vi "StageTest3.vi"() -> ()   [LabVIEW 2020]
uses:
  StageOptions.ctl
  SettingCtrlOptions.ctl
  PosCtrlOptions.ctl
  libximc.lvlib
  <instrlib>/_niInstr/Basic Elements/v1/FPGA/niInstr Basic Elements v1 FPGA.lvlib
panel:
  out "Y Maximum":dbl
  out "X Max Stage":dbl=220.0 format="%#_13g"
  in  "Move Step":dbl=1.0
  in  "Start Stage":bool
  in  "Speed Control (mm/s)":sgl(slide)=1.0 min=0.1 scale=0.1..5.0
  out "Y Step Size":sgl format="%#.2g"
  out "X Step Size":sgl format="%#.2g"
  in  "Scan Mode":enum16{"Raster", "Serpentine"}(ring)
  out "Controller Open?":bool
  in  "Y Position Abs":dbl caption="Y Position"
  in  "X Position Abs":dbl caption="X Position"
  in  "Move to Start":bool
  out "Move Step halved":dbl=1.0
  in  "Stop Stage":bool
  in  "Outline":bool
  in  "Stop Motion":bool
  in  "Right":bool
  in  "Left":bool
  in  "Down":bool
  in  "Up":bool
  in  "AbsMove":bool
  out "Moving?":bool
  in  "Zero":bool
  out "Y Position":dbl format="%#.3g"
  out "X Position":dbl format="%#.3g"
  out "Stage Position":cluster{sgl[], sgl[]}(graph) caption="XY Graph - Dark"
  in  "X Start":sgl
  in  "X End":sgl=10.0
  in  "Y Start":sgl
  in  "Y End":sgl=8.0
  in  "Y Step Size":sgl=0.5
  in  "X Step Size":sgl=0.5
  out "Line Count":i32=6
  out "Pixel Count":i32=6
  in  "Close Stage":bool
  in  "Machine Mode":T1(ring)=enum."Normal"
  out "Peripheral Coordis":sgl[][](array[numeric])=[[0.0, 0.0], [1.8, 0.0], [3.6, 0.0], [5.3999996, 0.0], [7.2, 0.0], [9.0, 0.0], [9.0, 2.0], [7.2, 2.0], [5.3999996, 2.0], [3.6, 2.0], [1.8, 2.0], [0.0, 2.0], [0.0, 4.0], [1.8, 4.0], [3.6, 4.0], [5.3999996, 4.0], [7.2, 4.0], [9.0, 4.0], [9.0, 6.0], [7.2, 6.0], [5.3999996, 6.0], [3.6, 6.0], [1.8, 6.0], [0.0, 6.0], [0.0, 8.0], [1.8, 8.0], [3.6, 8.0], [5.3999996, 8.0], [7.2, 8.0], [9.0, 8.0], [9.0, 10.0], [7.2, 10.0], [5.3999996, 10.0], [3.6, 10.0], [1.8, 10.0], [0.0, 10.0]]
  in  "Next Coordinate Index":i32
  out "Step Sizes":sgl[](array[numeric])
  out "Coordinate Array":sgl[][](array[numeric])
  out "IDs":i32[](array[numeric])
  out "Calibration":cluster{dbl, "MicrostepMode":u32}[](array[cluster])
  in  "EdgePt/nPixelMap":bool=TRUE
  in  "Correction Table Path (Hidden)":path
  out "Serial nos":u32[](array[numeric])
  out "Stage Status":T2
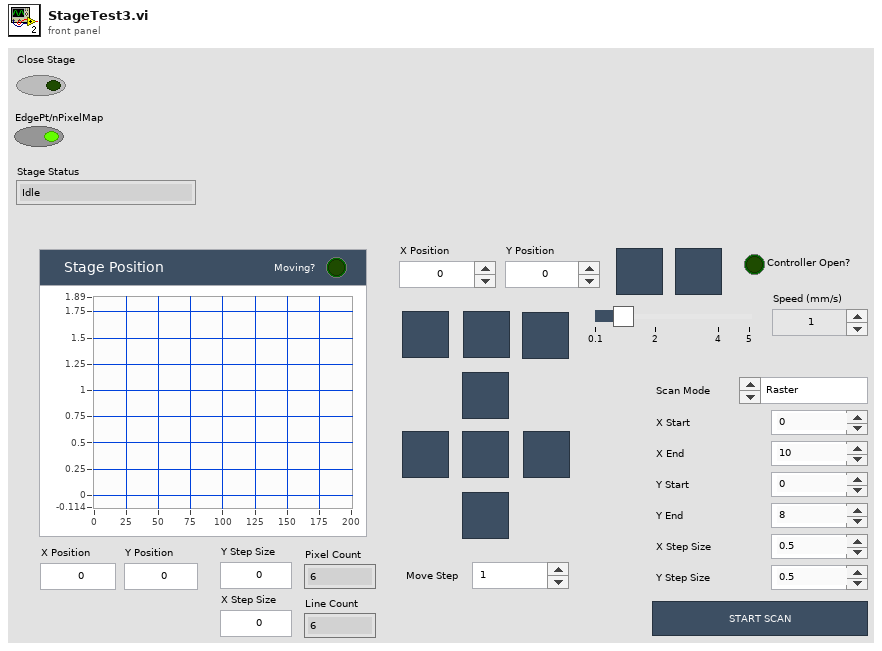
[diagram p1: front panel]
types:
  T1 = enum16{"Scanning Mode", "Perimeter Mode", "Normal"}
  T2 = typedef "StageOptions.ctl" = enum16{"Idle", "Init", "Set Speed", "GenerateMotionPoints", "Scan_Start", "Scan_MoveNext", "Scan_SyncSet", "Scan_Get Pos", "Scan_Complete", "Cmd_MoveAbs", "Cmd_CloseControllers", "Cmd_MoveUp", "Cmd_MoveDown", "Cmd_MoveLeft", "Cmd_MoveRight", "Cmd_MoveStart", "Cmd_MoveZero", "Cmd_GetPos", "Cmd_Stop", "Sync_On", "Sync_Off", "Stop Motion", "CloseApplication"}
  T3 = typedef "SettingCtrlOptions.ctl" = enum16{"Set X", "Set Y", "Set X and Y", "Get Settings", "None"}
  T4 = typedef "PosCtrlOptions.ctl" = enum16{"Move X", "Move Y", "Both X and Y", "Read Pos", "None"}
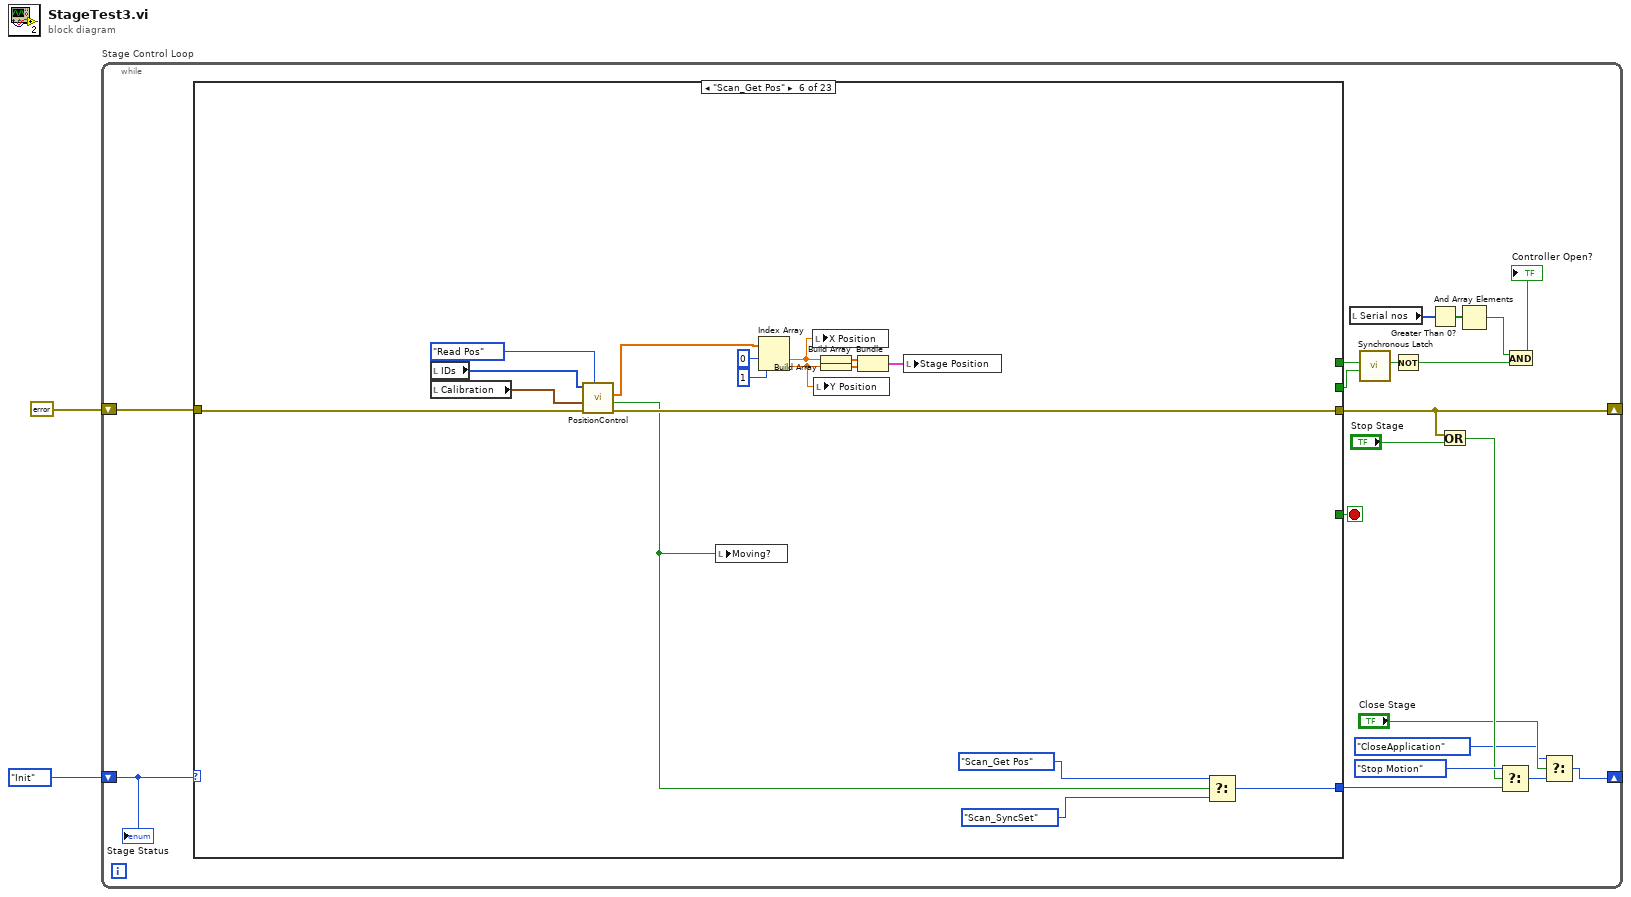
[diagram p0: block diagram]
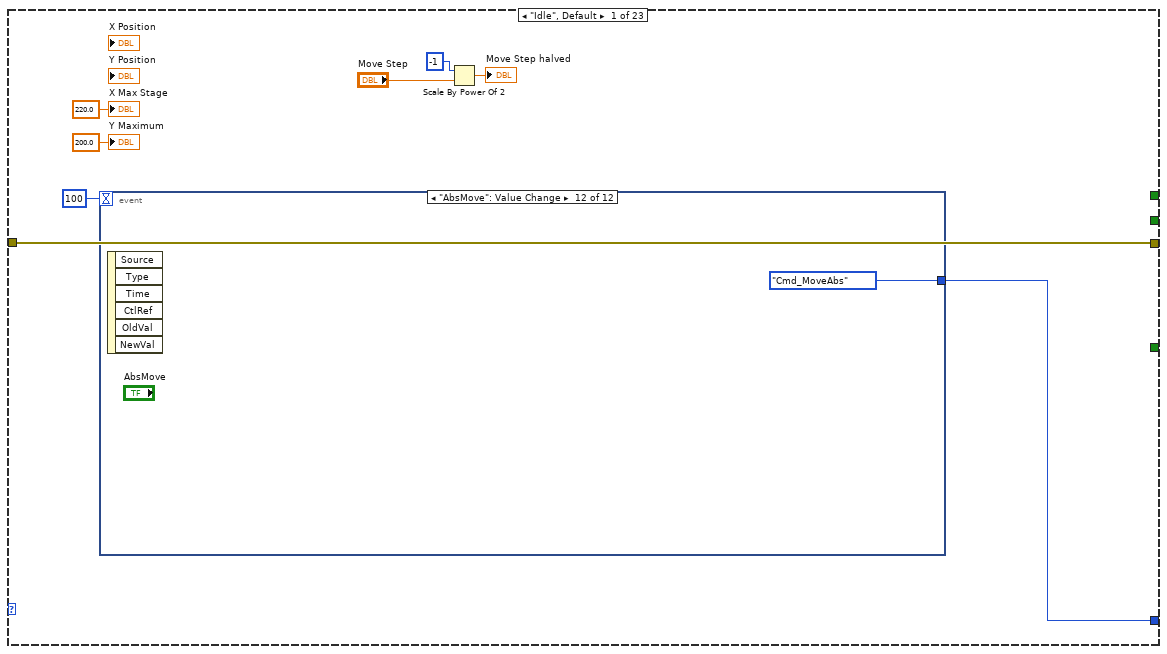
[diagram p2: hidden frame]
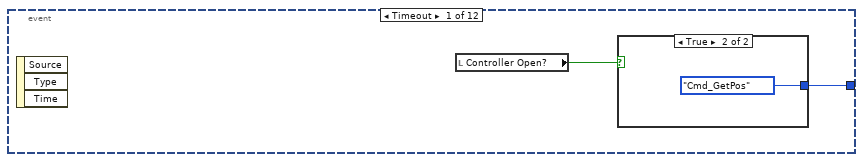
[diagram p3: hidden frame]
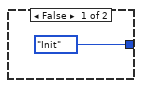
[diagram p4: hidden frame]
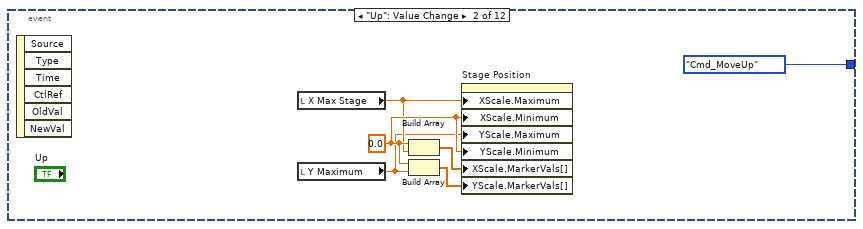
[diagram p5: hidden frame]
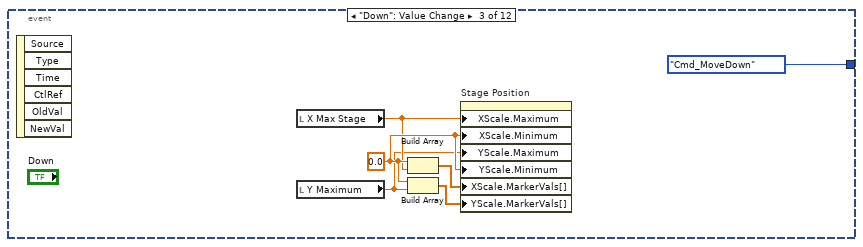
[diagram p6: hidden frame]
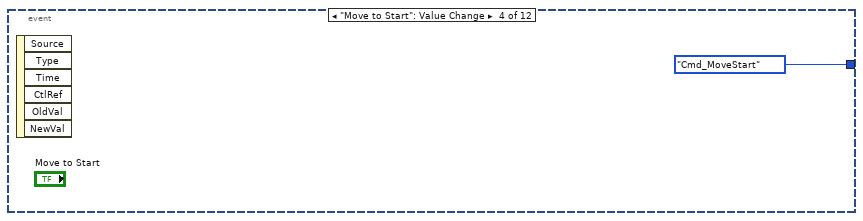
[diagram p7: hidden frame]
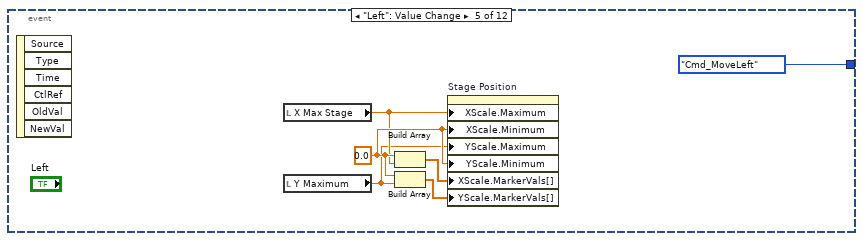
[diagram p8: hidden frame]
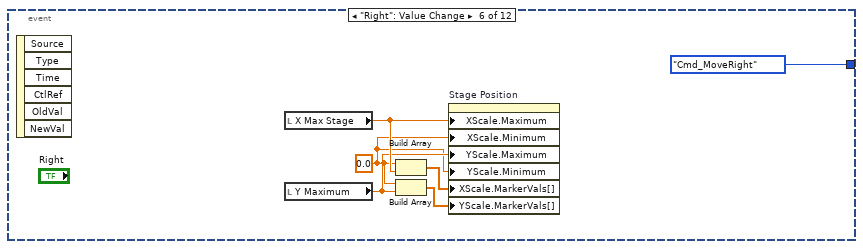
[diagram p9: hidden frame]
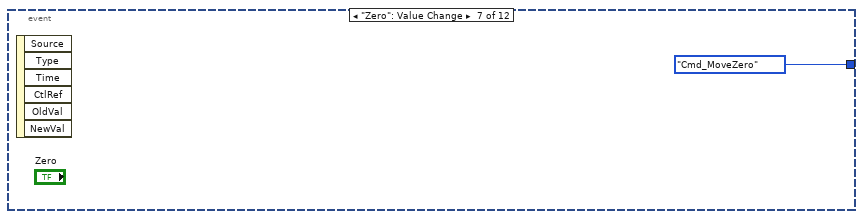
[diagram p10: hidden frame]
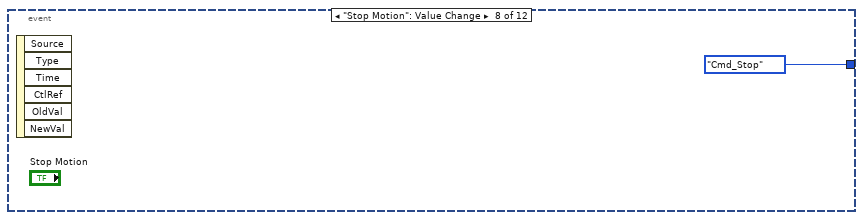
[diagram p11: hidden frame]
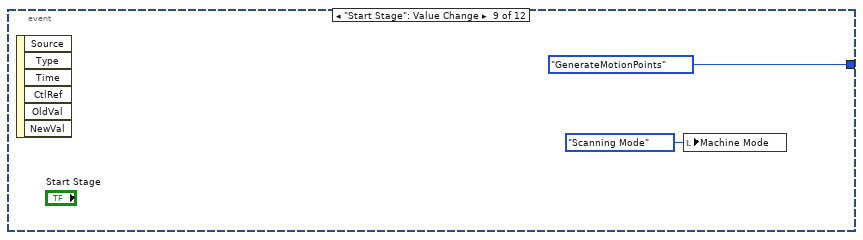
[diagram p12: hidden frame]
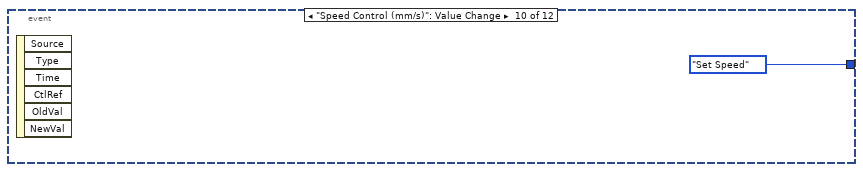
[diagram p13: hidden frame]
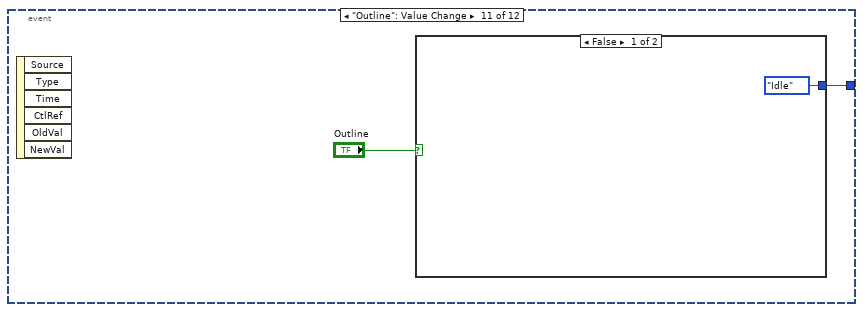
[diagram p14: hidden frame]
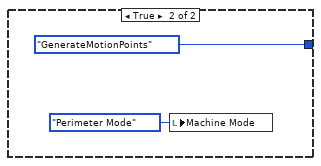
[diagram p15: hidden frame]
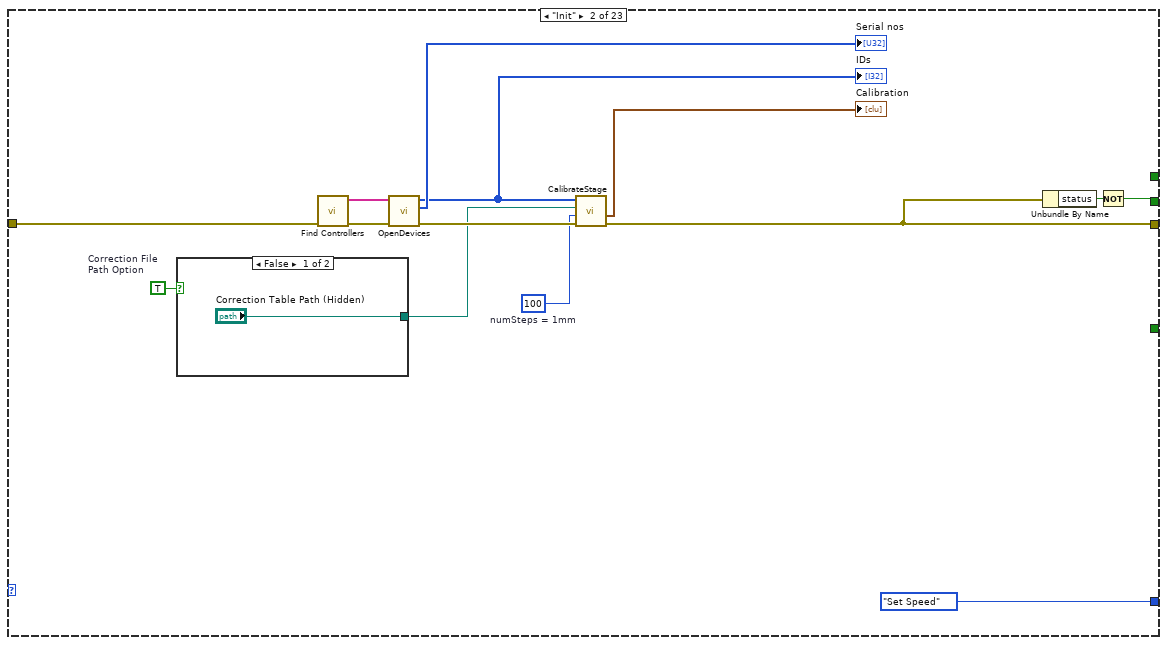
[diagram p16: hidden frame]
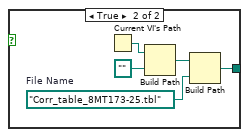
[diagram p17: hidden frame]
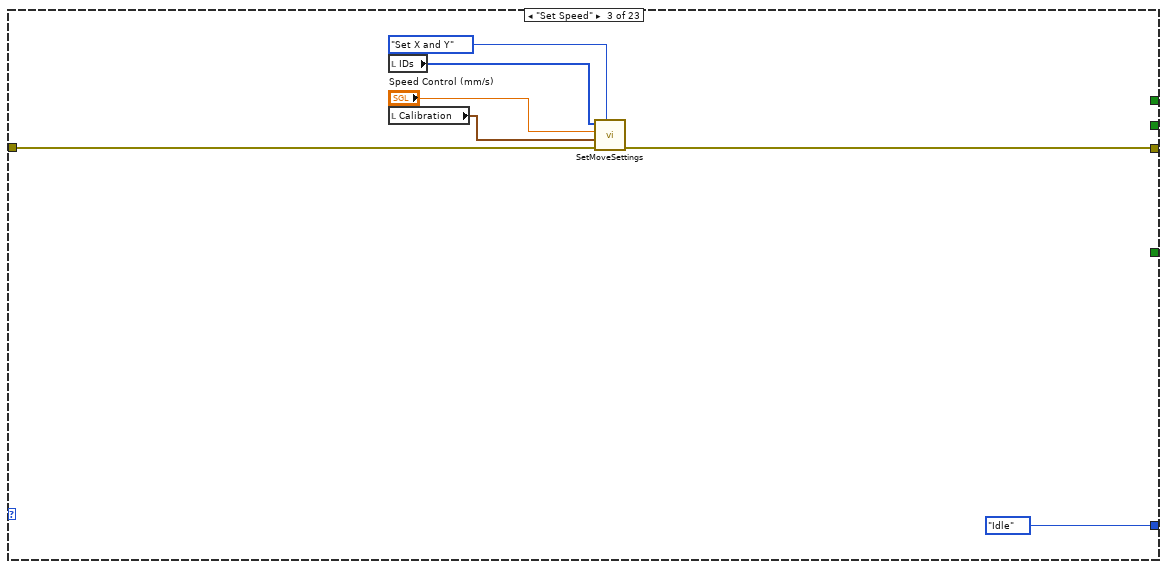
[diagram p18: hidden frame]
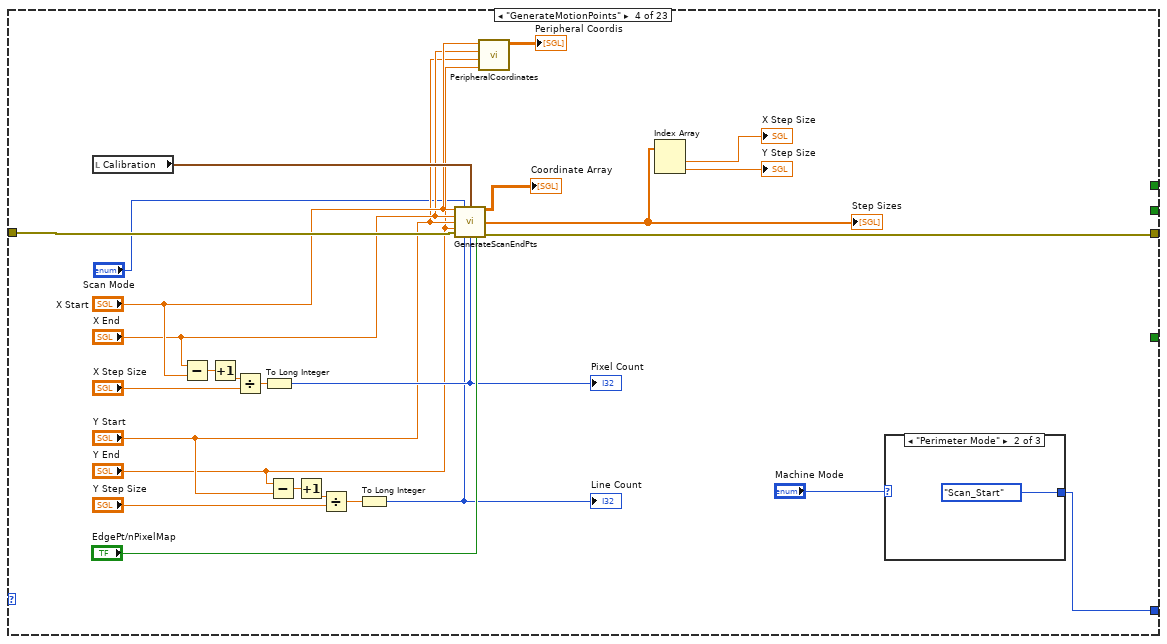
[diagram p19: hidden frame]
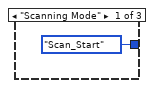
[diagram p20: hidden frame]
diagram:
  n1 = while "Stage Control Loop" {
    shift-right: [w11] -> _
    shift-left: StageOptions."Init" -> [w22]
    shift-right: [w19] -> _
    shift-left: errorcluster {"status"=FALSE, "code"=0, "source"=""} ("error out") -> [w20]
    stop <- w12 stop-if-true
    n2 = case shown="\"Scan_Get Pos\"" w22 {
      tunnel: [w30 w71 w94 w123 w137 w169 w183 w196 w237 w246 w255 w262 w273 w283 w293 w302 w310 w325 w331 w342 w351 w358 w368] -> w19
      tunnel: w20 -> [w30 w78 w95 w122 w143 w170 w184 w197 w238 w247 w256 w261 w274 w284 w294 w303 w311 w326 w330 w343 w352 w357 w367]
      tunnel: [w29 StageOptions."Set Speed" StageOptions."Idle" w103 StageOptions."Scan_Get Pos" w158 StageOptions."Scan_MoveNext" w193 StageOptions."Idle" StageOptions."Idle" StageOptions."Idle" StageOptions."Idle" StageOptions."Idle" StageOptions."Idle" StageOptions."Idle" StageOptions."Idle" StageOptions."Idle" StageOptions."Idle" StageOptions."Idle" StageOptions."Idle" StageOptions."Idle" StageOptions."Idle" StageOptions."Idle"] -> w17
      tunnel: [_ _ _ _ _ _ _ _ _ _ _ _ _ _ _ _ _ _ _ _ _ w354 w363] -> w15
      tunnel: [_ w72 _ _ _ _ _ _ _ _ _ _ _ _ _ _ _ _ _ _ _ _ _] -> w13
      tunnel: [_ _ _ _ _ _ _ _ _ _ _ _ _ _ _ _ _ _ _ _ _ _ w363] -> w12
      frame "Idle", Default {
        n3 = event shown="[11] \"AbsMove\": Value Change" {
          selector: _ -> [_ _ _ _ _ _ _ _ _ _ _ _]
          dyn-events: _ -> [_ _ _ _ _ _ _ _ _ _ _ _]
          timeout: 100 -> [_ _ _ _ _ _ _ _ _ _ _ _]
          tunnel: [w31 StageOptions."Cmd_MoveUp" StageOptions."Cmd_MoveDown" StageOptions."Cmd_MoveStart" StageOptions."Cmd_MoveLeft" StageOptions."Cmd_MoveRight" StageOptions."Cmd_MoveZero" StageOptions."Cmd_Stop" StageOptions."GenerateMotionPoints" StageOptions."Set Speed" w66 StageOptions."Cmd_MoveAbs"] -> w29
          event Timeout {
            n4 = event-data() -> ()  [unwired: 1 in, 3 out]
            n5 = local read "Controller Open?"() -> (w32:bool)
            n6 = case shown="True" w32 {
              tunnel: [StageOptions."Init" StageOptions."Cmd_GetPos"] -> w31
              frame False {
              }
              frame True {
              }
            }
          }
          event "Up": Value Change {
            w37 = 0.0 ("X Scale.Range:Minimum")
            n7 = event-data() -> ()  [unwired: 1 in, 6 out]
            n8 = local read "X Max Stage"() -> (w36:dbl)
            n9 = local read "Y Maximum"() -> (w35:dbl)
            n10 = Build Array(w37, w36) -> (w39:dbl[])
            n11 = Build Array(w37, w35) -> (w38:dbl[])
            n12 = property on="Stage Position" class="XYGraph (strict)"("XScale.Maximum"=w36, "XScale.Minimum"=w37, "YScale.Maximum"=w35, "YScale.Minimum"=w37, "XScale.MarkerVals[]"=w39, "YScale.MarkerVals[]"=w38) -> ()  [unwired: 2 in, 2 out]
          }
          event "Down": Value Change {
            w43 = 0.0 ("X Scale.Range:Minimum")
            n13 = event-data() -> ()  [unwired: 1 in, 6 out]
            n14 = local read "X Max Stage"() -> (w42:dbl)
            n15 = local read "Y Maximum"() -> (w41:dbl)
            n16 = Build Array(w43, w42) -> (w45:dbl[])
            n17 = Build Array(w43, w41) -> (w44:dbl[])
            n18 = property on="Stage Position" class="XYGraph (strict)"("XScale.Maximum"=w42, "XScale.Minimum"=w43, "YScale.Maximum"=w41, "YScale.Minimum"=w43, "XScale.MarkerVals[]"=w45, "YScale.MarkerVals[]"=w44) -> ()  [unwired: 2 in, 2 out]
          }
          event "Move to Start": Value Change {
            n19 = event-data() -> ()  [unwired: 1 in, 6 out]
          }
          event "Left": Value Change {
            w50 = 0.0 ("X Scale.Range:Minimum")
            n20 = event-data() -> ()  [unwired: 1 in, 6 out]
            n21 = local read "X Max Stage"() -> (w49:dbl)
            n22 = local read "Y Maximum"() -> (w48:dbl)
            n23 = Build Array(w50, w49) -> (w52:dbl[])
            n24 = Build Array(w50, w48) -> (w51:dbl[])
            n25 = property on="Stage Position" class="XYGraph (strict)"("XScale.Maximum"=w49, "XScale.Minimum"=w50, "YScale.Maximum"=w48, "YScale.Minimum"=w50, "XScale.MarkerVals[]"=w52, "YScale.MarkerVals[]"=w51) -> ()  [unwired: 2 in, 2 out]
          }
          event "Right": Value Change {
            w54 = 0.0 ("X Scale.Range:Minimum")
            n26 = event-data() -> ()  [unwired: 1 in, 6 out]
            n27 = local read "X Max Stage"() -> (w56:dbl)
            n28 = local read "Y Maximum"() -> (w55:dbl)
            n29 = Build Array(w54, w56) -> (w58:dbl[])
            n30 = Build Array(w54, w55) -> (w57:dbl[])
            n31 = property on="Stage Position" class="XYGraph (strict)"("XScale.Maximum"=w56, "XScale.Minimum"=w54, "YScale.Maximum"=w55, "YScale.Minimum"=w54, "XScale.MarkerVals[]"=w58, "YScale.MarkerVals[]"=w57) -> ()  [unwired: 2 in, 2 out]
          }
          event "Zero": Value Change {
            n32 = event-data() -> ()  [unwired: 1 in, 6 out]
          }
          event "Stop Motion": Value Change {
            n33 = event-data() -> ()  [unwired: 1 in, 6 out]
          }
          event "Start Stage": Value Change {
            n34 = event-data() -> ()  [unwired: 1 in, 6 out]
            n35 = local write "Machine Mode"(T1."Scanning Mode" ("Machine Mode")) -> ()
          }
          event "Speed Control (mm/s)": Value Change {
            n36 = event-data() -> ()  [unwired: 1 in, 6 out]
          }
          event "Outline": Value Change {
            n37 = event-data() -> ()  [unwired: 1 in, 6 out]
            n38 = case shown="False" "Outline" {
              tunnel: [StageOptions."Idle" StageOptions."GenerateMotionPoints"] -> w66
              frame False {
              }
              frame True {
                n39 = local write "Machine Mode"(T1."Perimeter Mode" ("Machine Mode")) -> ()
              }
            }
          }
          event "AbsMove": Value Change {
            n40 = event-data() -> ()  [unwired: 1 in, 6 out]
          }
        }
        n41 = Scale By Power Of 2(n=i16 -1, x="Move Step") -> (x*2^n=→"Move Step halved":dbl)
        "X Max Stage" <- 220.0 ("X Max Stage")
        "Y Maximum" <- 200.0 ("Y Maximum")
      }
      frame "Init" {
        w79 = 100  # numSteps = 1mm
        w80 = TRUE  # Correction File Path Option
        n42 = case shown="False" w80 {
          tunnel: ["Correction Table Path (Hidden)" w86] -> w81
          frame False {
          }
          frame True {
            w87 = path "Corr_table_8MT173-25.tbl"  # File Name
            n43 = Current VI's Path() -> (path=w89:path)
            n44 = Build Path(base path=w89, name or relative path=path "") -> (appended path=w88:path)
            n45 = Build Path(base path=w88, name or relative path=w87) -> (appended path=w86:path)
          }
        }
        n46 = call "Find Controllers.vi"("error in (no error)"=w78) -> ("error out"=w83:errorcluster, "Names"=w84:string[])  [unwired: 8 in, 1 out]
        n47 = call "OpenDevices.vi"("error In"=w83, "Names"=w84) -> ("error out"=w82:errorcluster, "Serial nos"=→"Serial nos":u32[], "IDs"=w76:i32[])  [unwired: 6 in]
        "IDs" <- w76
        n48 = call "CalibrateStage.vi"("error in (no error)"=w82, "numSteps = 1mm"=w79, "Correction Table Path"=w81, "IDs"=w76) -> ("error out"=w71:errorcluster, "Calibration"=→"Calibration":cluster{dbl, "MicrostepMode":u32}[])  [unwired: 2 in, 4 out]
        n49 = Unbundle By Name(w71) -> ("status"=w73:bool)
        n50 = Not(x=w73) -> (.not. x?=w72:bool)
      }
      frame "Set Speed" {
        n51 = local read "IDs"() -> (w93:i32[])
        n52 = local read "Calibration"() -> (w92:cluster{dbl, "MicrostepMode":u32}[])
        n53 = call "SetMoveSettings.vi"("Mode"=SettingCtrlOptions."Set X and Y", "error in (no error)"=w95, "Calibration"=w92, "Speed"="Speed Control (mm/s)", "IDs"=w93) -> ("error out"=w94:errorcluster)  [unwired: 4 in, 2 out]
      }
      frame "GenerateMotionPoints" {
        n54 = local read "Calibration"() -> (w109:cluster{dbl, "MicrostepMode":u32}[])
        n55 = Subtract(x="X End", y="X Start") -> (x-y=w119:sgl)
        n56 = Increment(x=w119) -> (x+1=w118:sgl)
        n57 = Divide(x=w118, y="X Step Size") -> (x/y=w116:sgl)
        n58 = To Long Integer(number=w116) -> (32bit integer=w115:i32)
        "Pixel Count" <- w115
        n59 = Subtract(x="Y End", y="Y Start") -> (x-y=w113:sgl)
        n60 = Increment(x=w113) -> (x+1=w114:sgl)
        n61 = Divide(x=w114, y="Y Step Size") -> (x/y=w111:sgl)
        n62 = To Long Integer(number=w111) -> (32bit integer=w110:i32)
        "Line Count" <- w110
        n63 = call "GenerateScanEndPts.vi"("X Start"="X Start", "Mode"="Scan Mode", "Calibration In"=w109, "X End"="X End", "Y Start"="Y Start", "Y End"="Y End", "error in"=w122, "Line Count"=w110, "Pixel Count"=w115, "EdgePt/nPixelMap"="EdgePt/nPixelMap") -> ("Coordinate Array"=→"Coordinate Array":sgl[][], "Step Sizes"=w100:sgl[], "error out"=w123:errorcluster)  [unwired: 3 in]
        "Step Sizes" <- w100
        n64 = call "PeripheralCoordinates.vi"("Y End"="Y End", "Y Start"="Y Start", "X End"="X End", "X Start"="X Start") -> ("Coordinate Array"=→"Peripheral Coordis":sgl[][])  [unwired: 7 in]
        n65 = Index Array(array=w100) -> (element #1=→"X Step Size":sgl, element #2=→"Y Step Size":sgl)  [unwired: 2 in]
        n66 = case shown="\"Perimeter Mode\"" "Machine Mode" {
          tunnel: [StageOptions."Scan_Start" StageOptions."Scan_Start" StageOptions."Idle"] -> w103
          frame "Scanning Mode" {
          }
          frame "Perimeter Mode" {
          }
          frame "Normal", Default {
          }
        }
      }
      frame "Scan_Start" {
        w140 = 0.0 ("element")
        w149 = 1.0  # Offset
        # "Draw Markers To Indicate the Scan Area"
        n67 = property on="X End" class="DigNum (strict)"() -> ("Value"=w148:sgl)  [unwired: 2 in, 2 out]
        n68 = property on="X Start" class="DigNum (strict)"() -> ("Value"=w147:sgl)  [unwired: 2 in, 2 out]
        n69 = property on="Y End" class="DigNum (strict)"() -> ("Value"=w144:sgl)  [unwired: 2 in, 2 out]
        n70 = property on="Y Start" class="DigNum (strict)"() -> ("Value"=w146:sgl)  [unwired: 2 in, 2 out]
        n71 = Add(x=w149, y=w148) -> (x+y=w151:dbl)
        n72 = Subtract(x=w147, y=w149) -> (x-y=w152:dbl)
        n73 = Add(x=w144, y=w149) -> (x+y=w150:dbl)
        n74 = Subtract(x=w146, y=w149) -> (x-y=w145:dbl)
        n75 = Build Array(w147, w148) -> (w154:sgl[])
        n76 = Build Array(w146, w144) -> (w153:sgl[])
        n77 = property on="Stage Position" class="XYGraph (strict)"(error in=w143, "XScale.Maximum"=w151, "XScale.Minimum"=w152, "YScale.Maximum"=w150, "YScale.Minimum"=w145, "XScale.MarkerVals[]"=w154, "YScale.MarkerVals[]"=w153) -> (error out=w129:errorcluster)  [unwired: 1 in, 1 out]
        n78 = local read "EdgePt/nPixelMap"() -> (w133:bool)
        n79 = local read "IDs"() -> (w136:i32[])
        n80 = local read "Step Sizes"() -> (w134:sgl[])
        n81 = local read "Calibration"() -> (w135:cluster{dbl, "MicrostepMode":u32}[])
        n82 = call "SetSyncSettings.vi"("Periodic/nPointScan"=w133, "X SyncOut Enabled"=FALSE, "Y SyncOut Enabled"=FALSE, "error in (no error)"=w129, "Calibration"=w135, "Step Sizes(mm)"=w134, "IDs"=w136) -> ("error out"=w130:errorcluster)  [unwired: 3 in, 1 out]
        n83 = local write "Next Coordinate Index"(0 ("Next Coordinate Index")) -> ()
        n84 = local read "IDs"() -> (w138:i32[])
        n85 = local read "Calibration"() -> (w139:cluster{dbl, "MicrostepMode":u32}[])
        n86 = Build Array(w140, w140) -> (w141:dbl[])
        n87 = call "PositionControlRelative.vi"("Mode"=PosCtrlOptions."Both X and Y", "error in (no error)"=w130, "Calibration"=w139, "Move to"=w141, "IDs"=w138) -> ("error out"=w137:errorcluster)  [unwired: 4 in, 2 out]
      }
      frame "Scan_Get Pos" {
        n88 = local read "IDs"() -> (w167:i32[])
        n89 = local read "Calibration"() -> (w168:cluster{dbl, "MicrostepMode":u32}[])
        n90 = call "PositionControl.vi"("Mode"=PosCtrlOptions."Read Pos", "error in (no error)"=w170, "Calibration"=w168, "IDs"=w167) -> ("error out"=w169:errorcluster, "Moving?"=w157:bool, "Position"=w160:sgl[])  [unwired: 4 in, 1 out]
        n91 = local write "Moving?"(w157) -> ()
        n92 = Index Array(array=w160, index #1=0 ("index"), index #2=1 ("index")) -> (element #1=w164:sgl, element #2=w163:sgl)
        n93 = local write "X Position"(w164) -> ()
        n94 = local write "Y Position"(w163) -> ()
        n95 = Build Array(w164) -> (w165:sgl[])
        n96 = Build Array(w163) -> (w166:sgl[])
        n97 = Bundle(w165, w166) -> (w159:cluster{sgl[], sgl[]})  [unwired: 1 in]
        n98 = local write "Stage Position"(w159) -> ()
        n99 = Select(t=StageOptions."Scan_Get Pos", s=w157, f=StageOptions."Scan_SyncSet") -> (s? t:f=w158:T2)
      }
      frame "Scan_SyncSet" {
        n100 = local read "EdgePt/nPixelMap"() -> (w173:bool)
        n101 = local read "IDs"() -> (w181:i32[])
        n102 = local read "Step Sizes"() -> (w179:sgl[])
        n103 = local read "Calibration"() -> (w180:cluster{dbl, "MicrostepMode":u32}[])
        n104 = Quotient & Remainder(x="Next Coordinate Index", y=2) -> (x-y*floor(x/y)=w176:i32)  [unwired: 1 out]
        n105 = Not Equal To 0?(x=w176) -> (x != 0?=w174:bool)
        n106 = Compound Arithmetic op=OR(invert w173, w174) -> (w175:bool)
        n107 = call "SetSyncSettings.vi"("Periodic/nPointScan"=w173, "X SyncOut Enabled"=w175, "Y SyncOut Enabled"=FALSE, "error in (no error)"=w184, "Calibration"=w180, "Step Sizes(mm)"=w179, "IDs"=w181) -> ("error out"=w183:errorcluster)  [unwired: 3 in, 1 out]
      }
      frame "Scan_MoveNext" {
        n108 = flat-sequence {
          tunnel: w197 -> [w200]
          tunnel: [w200] -> w188
          tunnel: [w199] -> w187
          tunnel: [w198] -> w185
          tunnel: [w208] -> w195
          tunnel: [w205] -> w194
          tunnel: [w204] -> w190
          tunnel: w188 -> [w209]
          tunnel: w187 -> [w204]
          tunnel: [w203] -> w186
          tunnel: w185 -> [w203]
          tunnel: [w219] -> w189
          tunnel: [w220] -> w196
          tunnel: w186 -> [w212]
          tunnel: w190 -> [w216]
          tunnel: w194 -> [w217]
          tunnel: w195 -> [w220]
          frame #0 {
            n109 = local read "Machine Mode"() -> (w198:T1)
            n110 = case shown="\"Perimeter Mode\"" w198 {
              tunnel: [w201 w202] -> w199
              frame "Scanning Mode", Default {
                n111 = local read "Coordinate Array"() -> (w201:sgl[][])
              }
              frame "Perimeter Mode" {
                n112 = local read "Peripheral Coordis"() -> (w202:sgl[][])
              }
            }
          }
          frame #1 {
            n113 = local read "IDs"() -> (w207:i32[])
            n114 = local read "Next Coordinate Index"() -> (w205:i32)
            n115 = local read "Calibration"() -> (w206:cluster{dbl, "MicrostepMode":u32}[])
            n116 = Index Array(array=w204, index (row)=w205) -> (element=w210:sgl[])  [unwired: 1 in]
            n117 = call "PositionControl.vi"("Mode"=PosCtrlOptions."Both X and Y", "error in (no error)"=w209, "Calibration"=w206, "Move to"=w210, "IDs"=w207) -> ("error out"=w208:errorcluster)  [unwired: 3 in, 3 out]
          }
          frame #2 {
            n118 = Matrix Size(0:w216) -> (1:w215:i32)  [unwired: 1 out]
            n119 = Increment(x=w217) -> (x+1=w213:i32)
            n120 = Greater?(x=w213, y=w215) -> (0:w214:bool)
            n121 = case shown="True" w214 {
              selector: w214 -> [w221 _]
              tunnel: w213 -> [w222 w225]
              tunnel: [w222 w224] -> w218
              tunnel: [w221 w223] -> w219
              tunnel: w212 -> [_ w226]
              frame False {
              }
              frame True {
                n122 = case shown="\"Scanning Mode\", Default" w226 {
                  tunnel: w225 -> [w228 _]
                  tunnel: [w228 0] -> w224
                  tunnel: [TRUE ("x > y?") w230] -> w223
                  frame "Scanning Mode", Default {
                  }
                  frame "Perimeter Mode" {
                    n123 = local read "Outline"() -> (w231:bool)
                    n124 = Not(x=w231) -> (.not. x?=w230:bool)
                  }
                }
              }
            }
            n125 = local write "Next Coordinate Index"(w218) -> ()
          }
        }
        n126 = Select(t=StageOptions."Scan_Complete", s=w189, f=StageOptions."Scan_Get Pos") -> (s? t:f=w193:T2)
      }
      frame "Scan_Complete" {
        w235 = 0.0 ("element")
        n127 = local read "IDs"() -> (w233:i32[])
        n128 = local read "Calibration"() -> (w234:cluster{dbl, "MicrostepMode":u32}[])
        n129 = Build Array(w235, w235) -> (w236:dbl[])
        n130 = call "PositionControl.vi"("Mode"=PosCtrlOptions."Both X and Y", "error in (no error)"=w238, "Calibration"=w234, "Move to"=w236, "IDs"=w233) -> ("error out"=w237:errorcluster)  [unwired: 3 in, 3 out]
      }
      frame "Cmd_MoveAbs" {
        n131 = local read "IDs"() -> (w245:i32[])
        n132 = local read "Calibration"() -> (w244:cluster{dbl, "MicrostepMode":u32}[])
        n133 = Build Array("X Position Abs", "Y Position Abs") -> (w243:dbl[])
        n134 = call "PositionControl.vi"("Mode"=PosCtrlOptions."Both X and Y", "error in (no error)"=w247, "Calibration"=w244, "Move to"=w243, "IDs"=w245) -> ("error out"=w246:errorcluster)  [unwired: 3 in, 3 out]
      }
      frame "Cmd_MoveStart" {
        n135 = local read "X Start"() -> (w250:sgl)
        n136 = local read "Y Start"() -> (w249:sgl)
        n137 = local read "IDs"() -> (w254:i32[])
        n138 = local read "Calibration"() -> (w253:cluster{dbl, "MicrostepMode":u32}[])
        n139 = Build Array(w250, w249) -> (w252:sgl[])
        n140 = call "PositionControl.vi"("Mode"=PosCtrlOptions."Both X and Y", "error in (no error)"=w256, "Calibration"=w253, "Move to"=w252, "IDs"=w254) -> ("error out"=w255:errorcluster)  [unwired: 3 in, 3 out]
      }
      frame "Cmd_CloseControllers" {
        n141 = local read "IDs"() -> (w259:i32[])
        n142 = for {
          shift-right: [w266] -> w263
          shift-left: w261 -> [w265]
          tunnel: w259 -> [w264] mode=indexing
          n143 = call "command stop.vi"("error in (no error)"=w265, "id"=w264) -> ("error out"=w266:errorcluster)  [unwired: 8 in, 1 out]
        }
        n144 = call "CloseDevices.vi"("error in (no error)"=w263, "Close"=TRUE, "Ids"=w259) -> ("error out"=w262:errorcluster)  [unwired: 8 in]
      }
      frame "Cmd_MoveUp" {
        n145 = local read "Move Step halved"() -> (w270:dbl)
        n146 = local read "IDs"() -> (w269:i32[])
        n147 = local read "Calibration"() -> (w268:cluster{dbl, "MicrostepMode":u32}[])
        n148 = Build Array(0.0 ("element"), w270) -> (w272:dbl[])
        n149 = call "PositionControlRelative.vi"("Mode"=PosCtrlOptions."Move Y", "error in (no error)"=w274, "Calibration"=w268, "Move to"=w272, "IDs"=w269) -> ("error out"=w273:errorcluster)  [unwired: 4 in, 2 out]
      }
      frame "Cmd_MoveDown" {
        n150 = local read "Move Step halved"() -> (w280:dbl)
        n151 = local read "IDs"() -> (w278:i32[])
        n152 = local read "Calibration"() -> (w277:cluster{dbl, "MicrostepMode":u32}[])
        n153 = Negate(x=w280) -> (-x=w279:dbl)
        n154 = Build Array(0.0 ("element"), w279) -> (w282:dbl[])
        n155 = call "PositionControlRelative.vi"("Mode"=PosCtrlOptions."Move Y", "error in (no error)"=w284, "Calibration"=w277, "Move to"=w282, "IDs"=w278) -> ("error out"=w283:errorcluster)  [unwired: 4 in, 2 out]
      }
      frame "Cmd_MoveLeft" {
        n156 = local read "Move Step halved"() -> (w291:dbl)
        n157 = local read "IDs"() -> (w287:i32[])
        n158 = local read "Calibration"() -> (w288:cluster{dbl, "MicrostepMode":u32}[])
        n159 = Negate(x=w291) -> (-x=w290:dbl)
        n160 = Build Array(w290, 0.0 ("element")) -> (w292:dbl[])
        n161 = call "PositionControlRelative.vi"("Mode"=PosCtrlOptions."Move X", "error in (no error)"=w294, "Calibration"=w288, "Move to"=w292, "IDs"=w287) -> ("error out"=w293:errorcluster)  [unwired: 4 in, 2 out]
      }
      frame "Cmd_MoveRight" {
        n162 = local read "Move Step halved"() -> (w300:dbl)
        n163 = local read "IDs"() -> (w298:i32[])
        n164 = local read "Calibration"() -> (w297:cluster{dbl, "MicrostepMode":u32}[])
        n165 = Build Array(w300, 0.0 ("element")) -> (w301:dbl[])
        n166 = call "PositionControlRelative.vi"("Mode"=PosCtrlOptions."Move X", "error in (no error)"=w303, "Calibration"=w297, "Move to"=w301, "IDs"=w298) -> ("error out"=w302:errorcluster)  [unwired: 4 in, 2 out]
      }
      frame "Cmd_MoveZero" {
        w308 = 0.0 ("element")
        n167 = local read "IDs"() -> (w306:i32[])
        n168 = local read "Calibration"() -> (w307:cluster{dbl, "MicrostepMode":u32}[])
        n169 = Build Array(w308, w308) -> (w309:dbl[])
        n170 = call "PositionControl.vi"("Mode"=PosCtrlOptions."Both X and Y", "error in (no error)"=w311, "Calibration"=w307, "Move to"=w309, "IDs"=w306) -> ("error out"=w310:errorcluster)  [unwired: 3 in, 3 out]
      }
      frame "Cmd_GetPos" {
        n171 = local read "IDs"() -> (w323:i32[])
        n172 = local read "Calibration"() -> (w324:cluster{dbl, "MicrostepMode":u32}[])
        n173 = call "PositionControl.vi"("Mode"=PosCtrlOptions."Read Pos", "error in (no error)"=w326, "Calibration"=w324, "IDs"=w323) -> ("error out"=w325:errorcluster, "Moving?"=→"Moving?":bool, "Position"=w315:sgl[])  [unwired: 4 in, 1 out]
        n174 = Index Array(array=w315, index #1=0 ("index"), index #2=1 ("index")) -> (element #1=w319:sgl, element #2=w318:sgl)
        n175 = local write "X Position"(w319) -> ()
        n176 = local write "Y Position"(w318) -> ()
        n177 = Build Array(w319) -> (w321:sgl[])
        n178 = Build Array(w318) -> (w322:sgl[])
        n179 = Bundle(w321, w322) -> (→"Stage Position":cluster{sgl[], sgl[]})  [unwired: 1 in]
      }
      frame "Cmd_Stop" {
        n180 = local read "IDs"() -> (w329:i32[])
        n181 = for {
          shift-right: [w334] -> w331
          shift-left: w330 -> [w333]
          tunnel: w329 -> [w332] mode=indexing
          n182 = call "command stop.vi"("error in (no error)"=w333, "id"=w332) -> ("error out"=w334:errorcluster)  [unwired: 8 in, 1 out]
        }
      }
      frame "Sync_On" {
        n183 = local read "EdgePt/nPixelMap"() -> (w337:bool)
        n184 = local read "IDs"() -> (w340:i32[])
        n185 = local read "Step Sizes"() -> (w338:sgl[])
        n186 = local read "Calibration"() -> (w339:cluster{dbl, "MicrostepMode":u32}[])
        n187 = call "SetSyncSettings.vi"("Periodic/nPointScan"=w337, "X SyncOut Enabled"=TRUE, "Y SyncOut Enabled"=FALSE, "error in (no error)"=w343, "Calibration"=w339, "Step Sizes(mm)"=w338, "IDs"=w340) -> ("error out"=w342:errorcluster)  [unwired: 3 in, 1 out]
      }
      frame "Sync_Off" {
        n188 = local read "EdgePt/nPixelMap"() -> (w346:bool)
        n189 = local read "IDs"() -> (w349:i32[])
        n190 = local read "Step Sizes"() -> (w347:sgl[])
        n191 = local read "Calibration"() -> (w348:cluster{dbl, "MicrostepMode":u32}[])
        n192 = call "SetSyncSettings.vi"("Periodic/nPointScan"=w346, "X SyncOut Enabled"=FALSE, "Y SyncOut Enabled"=FALSE, "error in (no error)"=w352, "Calibration"=w348, "Step Sizes(mm)"=w347, "IDs"=w349) -> ("error out"=w351:errorcluster)  [unwired: 3 in, 1 out]
      }
      frame "Stop Motion" {
        w354 = TRUE ("Close")
        n193 = local read "IDs"() -> (w356:i32[])
        n194 = for {
          shift-right: [w362] -> w359
          shift-left: w357 -> [w361]
          tunnel: w356 -> [w360] mode=indexing
          n195 = call "command stop.vi"("error in (no error)"=w361, "id"=w360) -> ("error out"=w362:errorcluster)  [unwired: 8 in, 1 out]
        }
        n196 = call "CloseDevices.vi"("error in (no error)"=w359, "Close"=w354, "Ids"=w356) -> ("error out"=w358:errorcluster)  [unwired: 8 in]
        n197 = local write "Moving?"(FALSE ("Moving?")) -> ()
      }
      frame "CloseApplication" {
        w363 = TRUE ("Close")
        n198 = local read "IDs"() -> (w366:i32[])
        n199 = for {
          shift-right: [w372] -> w369
          shift-left: w367 -> [w371]
          tunnel: w366 -> [w370] mode=indexing
          n200 = call "command stop.vi"("error in (no error)"=w371, "id"=w370) -> ("error out"=w372:errorcluster)  [unwired: 8 in, 1 out]
        }
        n201 = call "CloseDevices.vi"("error in (no error)"=w369, "Close"=w363, "Ids"=w366) -> ("error out"=w368:errorcluster)  [unwired: 8 in]
        n202 = local write "Moving?"(FALSE ("Moving?")) -> ()
      }
    }
    n203 = local read "Serial nos"() -> (w5:u32[])
    n204 = call <instrlib>:"Synchronous Latch.vi"("clear"=w13, "set"=w15) -> ("out"=w14:bool)  [unwired: 9 in]
    n205 = Not(x=w14) -> (.not. x?=w7:bool)
    n206 = Greater Than 0?(x=w5) -> (x > 0?=w4:bool[])
    n207 = Or(x=w19, y="Stop Stage") -> (x .or. y?=w16:bool)
    n208 = And Array Elements(Boolean array=w4) -> (logical AND=w3:bool)
    n209 = Select(t=StageOptions."Stop Motion", s=w16, f=w17) -> (s? t:f=w10:T2)
    n210 = And(x=w3, y=w7) -> (x .and. y?=→"Controller Open?":bool)
    n211 = Select(t=StageOptions."CloseApplication", s="Close Stage", f=w10) -> (s? t:f=w11:T2)
    "Stage Status" <- w22
  }
